vi "Create.vi"(8 "error in (no error)":errorcluster, 10 "Tolerance":dbl) -> (0 "error out":errorcluster, 3 "Tolerant Numeric Comparator Out":refnum<class "Tolerant Numeric Argument Comparator.lvclass">)   [LabVIEW 2020, in "Tolerant Numeric Argument Comparator.lvclass"]
uses:
  Tolerant Numeric Argument Comparator.lvclass
  Tolerant Numeric Argument Comparator.lvclass/Tolerant Numeric Argument Comparator.ctl
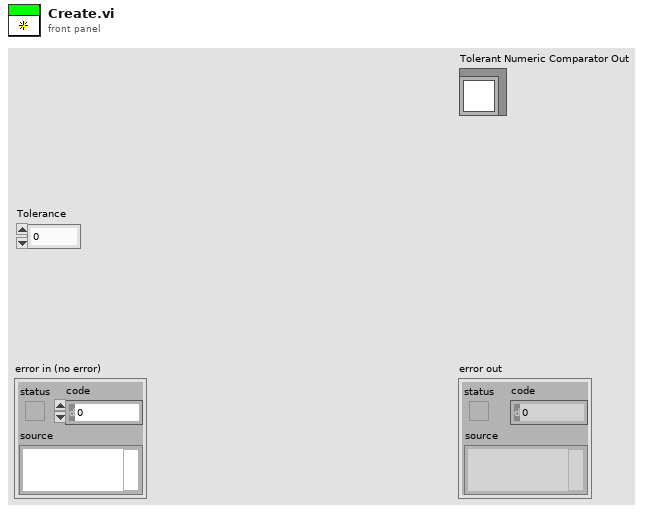
[diagram p1: front panel]
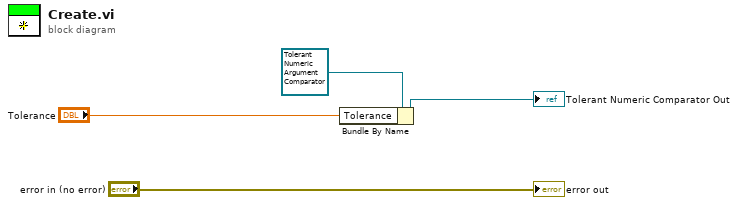
[diagram p0: block diagram]
diagram:
  n1 = Bundle By Name(cluster=refnum<class "Tolerant Numeric Argument Comparator.lvclass"> refnum ("Tolerant Numeric Comparator"), "Tolerance"="Tolerance") -> (→"Tolerant Numeric Comparator Out":refnum<class "Tolerant Numeric Argument Comparator.lvclass">)
  "error out" <- "error in (no error)"
